vi "Untitled 2.vi"() -> ()   [LabVIEW 2014]
panel:
  in  "Stop":bool
  out "Waveform Graph":dbl[](graph)
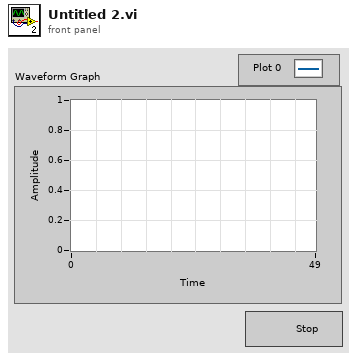
[diagram p1: front panel]
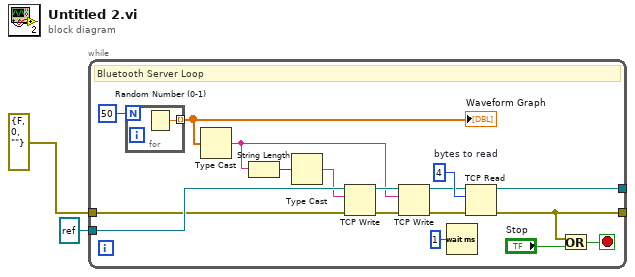
[diagram p0: block diagram]
diagram:
  n1 = while {
    tunnel: [w3] -> _
    tunnel: [w4] -> _
    tunnel: refnum<k31> refnum ("listener ID") -> [w19]
    tunnel: errorcluster {"status"=FALSE, "code"=0, "source"=""} ("error out") -> [w10]
    stop <- w12 stop-if-true
    w7 = 4  # bytes to read
    # "Bluetooth Server Loop"
    n2 = for {
      N: 50 ("# of Points") -> [_]
      tunnel: [w20] -> w8 mode=indexing
      n3 = Random Number (0-1)() -> (number: 0 to 1=w20:dbl)
    }
    "Waveform Graph" <- w8
    n4 = Type Cast(x=w8) -> (*(type *) &x=w14:string)  [unwired: 1 out]
    n5 = String Length(string=w14) -> (length=w16:i32)
    n6 = Type Cast(x=w16) -> (*(type *) &x=w15:string)  [unwired: 1 out]
    n7 = TCP Write(connection ID=w19, data in=w15, error in (no error)=w10) -> (connection ID out=w18:refnum<k31>, error out=w17:errorcluster)  [unwired: 2 out]
    n8 = TCP Write(connection ID=w18, data in=w14, error in (no error)=w17) -> (connection ID out=w6:refnum<k31>, error out=w5:errorcluster)  [unwired: 2 out]
    n9 = Wait (ms)(milliseconds to wait=u32 1) -> ()  [unwired: 1 out]
    n10 = TCP Read(connection ID=w6, bytes to read=w7, error in (no error)=w5) -> (connection ID out=w4:refnum<k31>, error out=w3:errorcluster)  [unwired: 3 out]
    n11 = Or(x=w3, y="Stop") -> (x .or. y?=w12:bool)
  }
